vi "sub_log_fine-name.vi"() -> ()   [LabVIEW 2019]
uses:
  logfile-name.vi
panel:
  out "custome time log-name":string
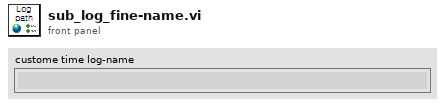
[diagram p1: front panel]
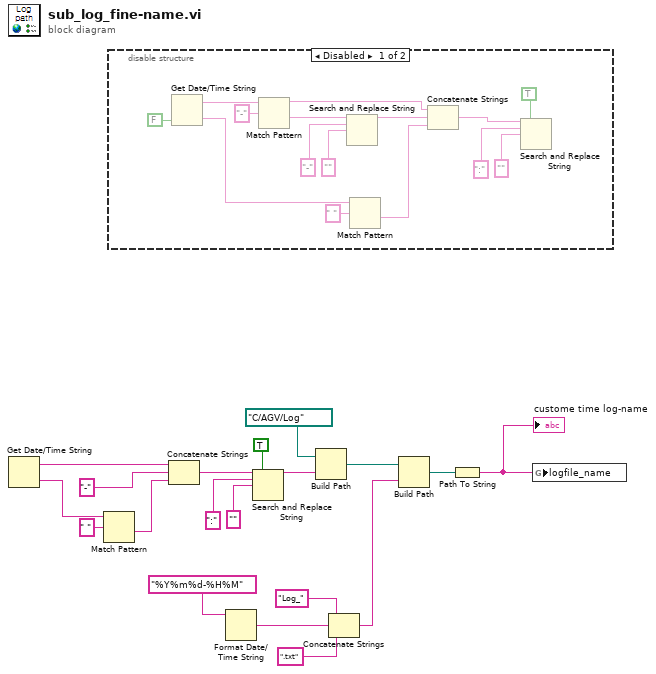
[diagram p0: block diagram]
diagram:
  n1 = Get Date/Time String() -> (date string=w7:string, time string=w13:string)  [unwired: 3 in]
  n2 = Match Pattern(string=w13, regular expression=" " ("정규식")) -> (after substring=w12:string)  [unwired: 1 in, 3 out]
  n3 = disable-structure shown="Disabled" {
    frame Disabled {
      n4 = Get Date/Time String(want seconds? (F)=FALSE ("초 보이기? (거짓)")) -> (date string=w29:string, time string=w26:string)  [unwired: 2 in]
      n5 = Match Pattern(string=w29, regular expression="-" ("정규식")) -> (before substring=w20:string, after substring=w24:string)  [unwired: 1 in, 2 out]
      n6 = Search and Replace String(input string=w24, search string="-" ("검색 문자열"), replace string="" ("대체 문자열(\"\")")) -> (result string=w21:string)  [unwired: 5 in, 3 out]
      n7 = Match Pattern(string=w26, regular expression=" " ("정규식")) -> (after substring=w25:string)  [unwired: 1 in, 3 out]
      n8 = Concatenate Strings(w20, w21, w25) -> (w34:string)
      n9 = Search and Replace String(replace all?=TRUE ("모두 대체? (거짓)"), input string=w34, search string=":" ("검색 문자열"), replace string="" ("대체 문자열(\"\")")) -> ()  [unwired: 4 in, 4 out]
    }
    frame Enabled {
    }
  }
  n10 = Concatenate Strings(w7, "-" ("정규식"), w12) -> (w8:string)
  n11 = Format Date/Time String(time format string (%c)="%Y%m%d-%H%M") -> (date/time string=w16:string)  [unwired: 2 in]
  n12 = Search and Replace String(replace all?=TRUE ("모두 대체? (거짓)"), input string=w8, search string=":" ("검색 문자열"), replace string="" ("대체 문자열(\"\")")) -> (result string=w5:string)  [unwired: 4 in, 3 out]
  n13 = Build Path(base path=path "C:/AGV/Log" ("베이스 경로"), name or relative path=w5) -> (appended path=w3:path)
  n14 = Concatenate Strings("Log_", w16, ".txt" ("문자열")) -> (w4:string)
  n15 = Build Path(base path=w3, name or relative path=w4) -> (appended path=w2:path)
  n16 = Path To String(path=w2) -> (string=w1:string)
  "custome time log-name" <- w1
  n17 = global write "logfile-name.vi" "logfile_name"(w1) -> ()
